vi "去掉第一个节点.vi"(10 "Xml Node Name":string, 11 "XML String In":string) -> (3 "XML String Out":string)   [LabVIEW 2014]
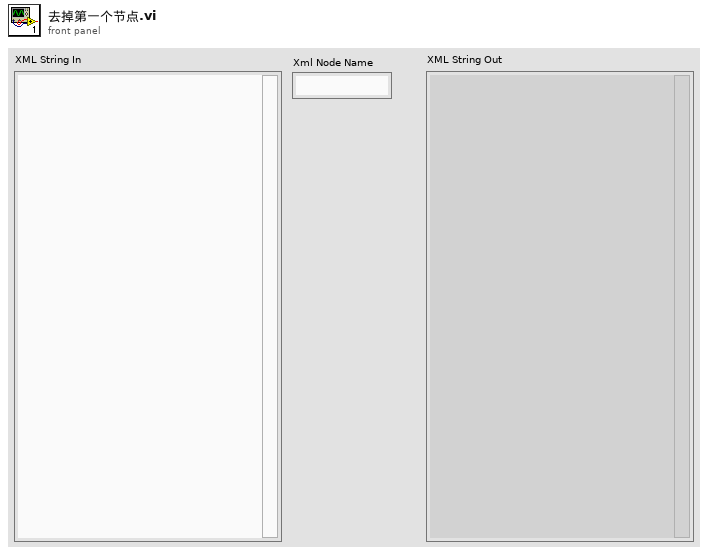
[diagram p1: front panel]
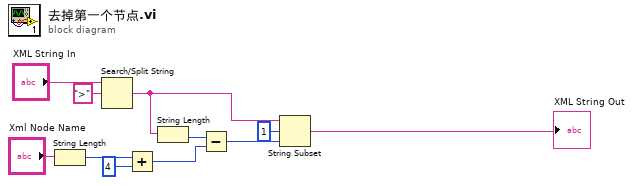
[diagram p0: block diagram]
diagram:
  n1 = String Length(string="Xml Node Name") -> (length=w3:i32)
  n2 = Search/Split String(string="XML String In", search string/char (-)=">" ("搜索字符串/字符(-)")) -> (match + rest of string=w8:string)  [unwired: 1 in, 2 out]
  n3 = Add(x=w3, y=4) -> (x+y=w2:i32)
  n4 = String Length(string=w8) -> (length=w9:i32)
  n5 = Subtract(x=w9, y=w2) -> (x-y=w5:i32)
  n6 = String Subset(string=w8, offset (0)=1 ("偏移量(0)"), length (rest)=w5) -> (substring=→"XML String Out":string)
